vi "AlliGator Python Plugin Data to Graph v1.1.vi"(7 "AlliGator Ctrl Refnums":T8, 8 "error in (no error)":errorcluster, 10 "Output Destination":string, 11 "Plugin_Data":T1) -> (0 "error out":errorcluster, 3 "Message":string)   [LabVIEW 2021, in "AlliGator Python Plugins.lvlib"]
uses:
  AlliGator Python Plugins.lvlib
  Strings/Strings.lvlib
  GUI/AlliGator GUI.lvlib
  Graphs/XY Graph/XY Graph Add-Ons.lvlib
  GUI/AlliGator Registered Events Ctrl Refnums.ctl
  Source Image/AlliGator Displayed Image.ctl
  Source Image/AlliGator Source Image.lvlib
  GUI/AlliGator Dataset Ctrl Refnums.ctl
  Phasor/Phasor Calibration Type.ctl
  Phasor/Phasor.lvlib
  GUI/AlliGator Phasor Graph Ctrl Refnums.ctl
  GUI/AlliGator Phasor Plot Ctrl Refnums.ctl
  GUI/AlliGator State Indicator.ctl
  GUI/AlliGator Main Window Tabs.ctl
  GUI/AlliGator Other Ctrl Refnums.ctl
  Histograms/Histogram Bin Position.ctl
  Histograms/Histogram Window.lvlib
  Histograms/Histogram Bin Option.ctl
  Histograms/Linear Histogram Options.ctl
  GUI/AlliGator Image Histogram Control Refnums.ctl
  Fits/IRF(X)PSED/Decay Fit Parameters & Derived Quantities List v2.ctl
  Fits/Fits.lvlib
  Decay Fit Parameter Map/AlliGator Decay Fit Map Control Refnums.ctl
  Decay Fit Parameter Map/AlliGator Decay Fit Parameter Map.lvlib
  Parameter Map/AlliGator Parameter Map Control Refnums.ctl
  Parameter Map/AlliGator Parameter Map.lvlib
  GUI/AlliGator Ctrl Refnums.ctl
  API v1/AlliGator Python Plugin Image Data v1.ctl
  AlliGator Python Plugin FLI Dataset Data v1.1.ctl
  Image/Image Point.ctl
  Image/Image.lvlib
  AlliGator Python Plugin Parameter Map Data v1.1.ctl
  API v1/AlliGator Python Plugin Plot Data v1.ctl
  API v1/AlliGator Python Plugin Graph Data v1.ctl
  AlliGator Python Plugin Data v1.1.ctl
panel:
  # "see the License on the block diagram (Ctrl+E or Window:Show Block Diagram)"
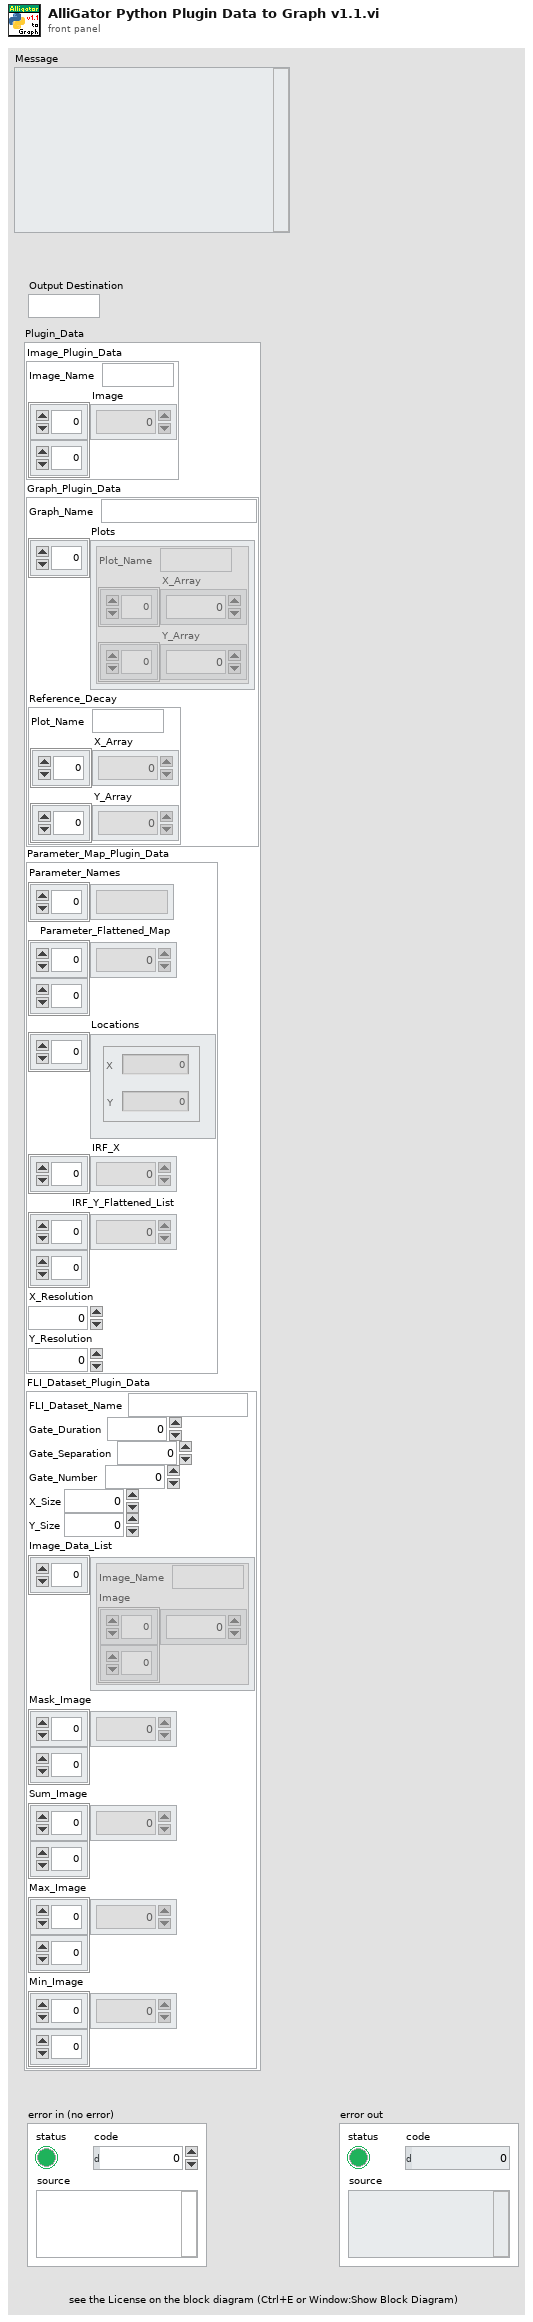
[diagram p1: front panel]
types:
  T1 = typedef "AlliGator Python Plugins.lvlib/AlliGator Python Plugin Data v1.1.ctl" = cluster{"Image_Plugin_Data":T2, "Graph_Plugin_Data":T3, "Parameter_Map_Plugin_Data":T5, "FLI_Dataset_Plugin_Data":T7}
  T2 = typedef "AlliGator Python Plugins.lvlib/AlliGator Python Plugin Image Data v1.ctl" = cluster{"Image_Name":string, "Image":sgl[][]}
  T3 = typedef "AlliGator Python Plugins.lvlib/AlliGator Python Plugin Graph Data v1.ctl" = cluster{"Graph_Name":string, "Plots":T4[], "Reference_Decay":T4}
  T4 = typedef "AlliGator Python Plugins.lvlib/AlliGator Python Plugin Plot Data v1.ctl" = cluster{"Plot_Name":string, "X_Array":dbl[], "Y_Array":dbl[]}
  T5 = typedef "AlliGator Python Plugins.lvlib/AlliGator Python Plugin Parameter Map Data v1.1.ctl" = cluster{"Parameter_Names":string[], "Parameter_Flattened_Map":dbl[][], "Locations":T6[], "IRF_X":dbl[], "IRF_Y_Flattened_List":dbl[][], "X_Resolution":i32, "Y_Resolution":i32}
  T6 = typedef "Image.lvlib/Image Point.ctl" = cluster{"X":i32, "Y":i32}
  T7 = typedef "AlliGator Python Plugins.lvlib/AlliGator Python Plugin FLI Dataset Data v1.1.ctl" = cluster{"FLI_Dataset_Name":string, "Gate_Duration":dbl, "Gate_Separation":dbl, "Gate_Number":i32, "X_Size":i32, "Y_Size":i32, "Image_Data_List":T2[], "Mask_Image":u16[][], "Sum_Image":sgl[][], "Max_Image":sgl[][], "Min_Image":sgl[][]}
  T8 = typedef "AlliGator GUI.lvlib/AlliGator Ctrl Refnums.ctl" = cluster{"Other AlliGator Ctrl Refnums":T9, "Phasor Plot Ctrl Refnums":T10, "Phasor Graph Ctrl Refnums":T11, "Dataset Control Refnums":T12, "Registered Events Ctrl Refnums":T13, "Image Histogram Ctrl Refnums":T14, "Decay Fit Map Ctrl Refnums":T15, "Parameter Map Ctrl Refnums":T16}
  T9 = typedef "AlliGator GUI.lvlib/AlliGator Other Ctrl Refnums.ctl" = cluster{"State Indicators":refnum<vi>, " Progress Bar":refnum<vi>, "Decay Graph Active":refnum<vi>, "Decay Statistics Bin":refnum<vi>, "Time Step":refnum<vi>, "Use File Timestamp":refnum<vi>, "Tab Control":refnum<vi>, "CPU":refnum<vi>, "Abort Fit":refnum<vi>, "Dataset File/Folder Path":refnum<vi>, "Abort ROI Creation":refnum<vi>, "Event LED":refnum<vi>, "Dataset File/Folder Path 2":refnum<vi>, "Dataset File/Folder Path 3":refnum<vi>, "Dataset File/Folder Path 4":refnum<vi>, "Dataset File/Folder Path 5":refnum<vi>, "Dataset File/Folder Path 6":refnum<vi>, "Dataset File/Folder Path 7":refnum<vi>, "Dataset File/Folder Path 8":refnum<vi>, "Dataset File/Folder Path 9":refnum<vi>, "Dataset File/Folder Path 10":refnum<vi>, "Dataset File/Folder Path 11":refnum<vi>}
  T10 = typedef "AlliGator GUI.lvlib/AlliGator Phasor Plot Ctrl Refnums.ctl" = cluster{"Phasor Ratio":refnum<vi>, "Modulus Lifetime":refnum<vi>, "Phasor at cursor (m, phi)":refnum<vi>, "Phase Lifetime":refnum<vi>, "Phasor at cursor (g, s)":refnum<vi>, "Phasor Plor Average Lifetime":refnum<vi>, "Phasor Plot Active":refnum<vi>, "Save Phasor Plot":refnum<vi>, "Image Overlay Color":refnum<vi>, "Phasor Plot Color Scale":refnum<vi>, "Reference 1 Button":refnum<vi>, "Reference 2 Button":refnum<vi>, "True Phasor Plot Value":refnum<vi>}
  T11 = typedef "AlliGator GUI.lvlib/AlliGator Phasor Graph Ctrl Refnums.ctl" = cluster{"Phasor Ratio":refnum<vi>, "Modulus Lifetime":refnum<vi>, "Phasor at cursor (m, phi)":refnum<vi>, "Phase Lifetime":refnum<vi>, "Phasor at cursor (g, s)":refnum<vi>, "Phasor Graph Average Lifetime":refnum<vi>, "Phasor Graph Active":refnum<vi>, "Save Phasor Graph":refnum<vi>, "Phasor Frame Slide":refnum<vi>, "Single Step Phasor":refnum<vi>, "Calibration Type":refnum<vi>, "Show Line":refnum<vi>, "Phase Lifetime 1":refnum<vi>, "Phase Lifetime 2":refnum<vi>, "Phasor Graph Frequency":refnum<vi>, "Phasor Reference 1 Control":refnum<vi>, "Phasor Reference 2 Control":refnum<vi>, "Calibration Lifetime":refnum<vi>, "Phase Lifetime SDV":refnum<vi>, "Average Lifetime SDV":refnum<vi>, "Phasor Ratio SDV":refnum<vi>, "Modulus Lifetime SDV":refnum<vi>}
  T12 = typedef "AlliGator GUI.lvlib/AlliGator Dataset Ctrl Refnums.ctl" = cluster{"Current Data":refnum<vi>, "Gate Image Slide":refnum<vi>, "Time Point Slide":refnum<vi>, "Current Time Stamp":refnum<vi>, "Save Image":refnum<vi>, "Displayed Image":refnum<vi>, "Overlay Mode":refnum<vi>, "Phasor Overlay Color":refnum<vi>, "Image Color Scale":refnum<vi>, "Use ROI as Search Area":refnum<vi>, "Source Image ROI Color":refnum<vi>, "True Pixel Value":refnum<vi>}
  T13 = typedef "AlliGator GUI.lvlib/AlliGator Registered Events Ctrl Refnums.ctl" = cluster{"Time Point Slider":refnum<vi>, "Phasor Plot Display Range":refnum<vi>, "Decay Graph":refnum<vi>, "Decay Statistics Graph":refnum<vi>, "Intensity Time Trace":refnum<vi>, "Phasor Graph":refnum<vi>, "Phasor Ratio Graph":refnum<vi>, "Lifetime Graph":refnum<vi>, "Phasor Plot Display":refnum<vi>, "Source Image Display":refnum<vi>, "Decay Fit Parameter Map Display Range":refnum<vi>, "Decay Fit Parameter Map Display":refnum<vi>, "Parameter Map Display Range":refnum<vi>, "Parameter Map Display":refnum<vi>, "Phasor Plot Display Range":refnum<vi>}
  T14 = typedef "AlliGator GUI.lvlib/AlliGator Image Histogram Control Refnums.ctl" = cluster{"Image Histogram":refnum<vi>, "Image Histogram Options":refnum<vi>, "Image Histogram Active":refnum<vi>, "Image Histogram Upper Percentile":refnum<vi>, "Image Histogram Lower Percentile":refnum<vi>, "Auto-Adjust Contrast":refnum<vi>}
  T15 = typedef "AlliGator Decay Fit Parameter Map.lvlib/AlliGator Decay Fit Map Control Refnums.ctl" = cluster{"Decay Fit Parameter Map Color Scale":refnum<vi>, "Decay Fit Parameter":refnum<vi>, "Max Parameter":refnum<vi>, "Min Parameter":refnum<vi>, "Decay Fit Parameter Map Display":refnum<vi>, "Decay Fit Parameter Map Display Range":refnum<vi>, "Decay Parameter Map X":refnum<vi>, "Decay Parameter Map Y":refnum<vi>, "Decay Parameter Map Value":refnum<vi>}
  T16 = typedef "AlliGator Parameter Map.lvlib/AlliGator Parameter Map Control Refnums.ctl" = cluster{"Parameter Map Color Scale":refnum<vi>, "Map Parameter":refnum<vi>, "Max Parameter":refnum<vi>, "Min Parameter":refnum<vi>, "Parameter Map Display":refnum<vi>, "Parameter Map Display Range":refnum<vi>, "Parameter Map Set":refnum<vi>, "Parameter Map X":refnum<vi>, "Parameter Map Y":refnum<vi>, "Parameter Map Value":refnum<vi>}
  T17 = typedef "XY Graph Add-Ons.lvlib/XY Graph Refnum.ctl" = refnum<vi>
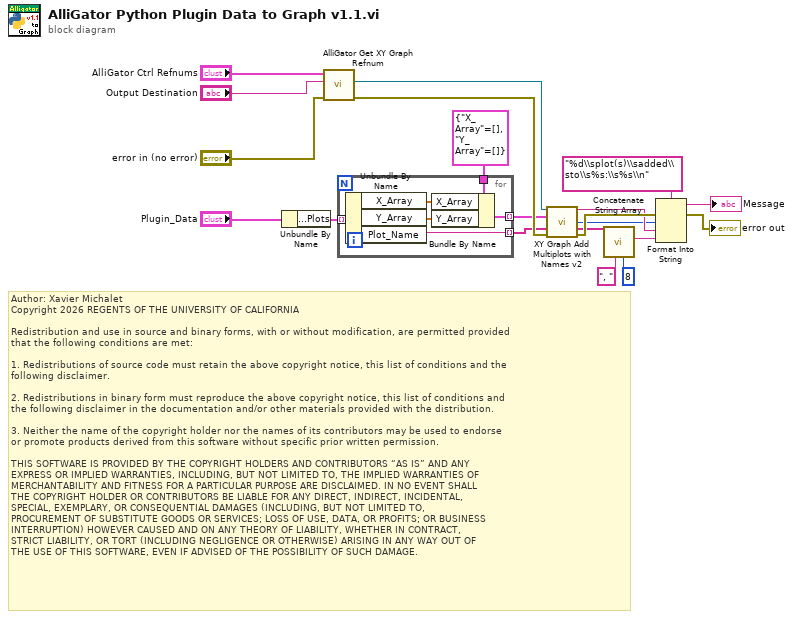
[diagram p0: block diagram]
diagram:
  # "Author: Xavier Michalet\nCopyright 2026 REGENTS OF THE UNIVERSITY OF CALIFORNIA\n\nRedistribution and use in source and binary forms, with or without modification, are permitted provided\nthat the following conditions are met:\n\n1. Redistributions of source code must retain the above copyright notice, this list of conditions and the\nfollowing disclaimer.\n\n2. Redistributions in binary form must reproduce the above copyright notice, this list of conditions and\nthe following disclaimer in the documentation and/or other materials provided with the distribution.\n\n3. Neither the name of the copyright holder nor the names of its contributors may be used to endorse \nor promote products derived from this software without specific prior written permission.\n\nTHIS SOFTWARE IS PROVIDED BY THE COPYRIGHT HOLDERS AND CONTRIBUTORS “AS IS” AND ANY \nEXPRESS OR IMPLIED WARRANTIES, INCLUDING, BUT NOT LIMITED TO, THE IMPLIED WARRANTIES OF\nMERCHANTABILITY AND FITNESS FOR A PARTICULAR PURPOSE ARE DISCLAIMED. IN NO EVENT SHALL\nTHE COPYRIGHT HOLDER OR CONTRIBUTORS BE LIABLE FOR ANY DIRECT, INDIRECT, INCIDENTAL, \nSPECIAL, EXEMPLARY, OR CONSEQUENTIAL DAMAGES (INCLUDING, BUT NOT LIMITED TO, \nPROCUREMENT OF SUBSTITUTE GOODS OR SERVICES; LOSS OF USE, DATA, OR PROFITS; OR BUSINESS\nINTERRUPTION) HOWEVER CAUSED AND ON ANY THEORY OF LIABILITY, WHETHER IN CONTRACT, \nSTRICT LIABILITY, OR TORT (INCLUDING NEGLIGENCE OR OTHERWISE) ARISING IN ANY WAY OUT OF\nTHE USE OF THIS SOFTWARE, EVEN IF ADVISED OF THE POSSIBILITY OF SUCH DAMAGE."
  n1 = Unbundle By Name("Plugin_Data") -> ("Graph_Plugin_Data.Plots"=w8:T4[])
  n2 = call "AlliGator Get XY Graph Refnum.vi"("error in (no error)"="error in (no error)", "XY Graph Name"="Output Destination", "AlliGator Ctrl Refnums"="AlliGator Ctrl Refnums") -> ("error out"=w17:errorcluster, "XY Graph reference"=w19:T17)  [unwired: 7 in]
  n3 = for {
    tunnel: w8 -> [w26] mode=indexing
    tunnel: [w25] -> w3 mode=indexing
    tunnel: cluster{"X_Array":dbl[], "Y_Array":dbl[]} {"X_Array"=[], "Y_Array"=[]} -> [w23]
    tunnel: [w21] -> w2 mode=indexing
    n4 = Unbundle By Name(w26) -> ("X_Array"=w24:dbl[], "Y_Array"=w22:dbl[], "Plot_Name"=w25:string)
    n5 = Bundle By Name(cluster=w23, "X_Array"=w24, "Y_Array"=w22) -> (w21:cluster{"X_Array":dbl[], "Y_Array":dbl[]})
  }
  n6 = call "XY Graph Add Multiplots with Names v2.vi"("XYGraph in"=w19, "Array of Plots"=w2, "Array of Plot Names (\"Plot\")"=w3, "error in (no error)"=w17) -> ("XY Graph Caption (or Label)"=w11:string, "Number of Plots Added"=w10:i32, "Added Plot Names"=w4:string[], "error out"=w13:errorcluster)  [unwired: 7 in, 1 out]
  n7 = call "Concatenate String Array.vi"("Max Number of Elements (None: -1)"=8, "Separator (TAB)"=", ", "String Array"=w4) -> ("Formatted String"=w12:string)  [unwired: 8 in]
  n8 = Format Into String(format string="%d\\splot(s)\\sadded\\sto\\s%s:\\s%s\\n", error in=w13, w10, w11, w12) -> (resulting string=→"Message":string, error out=→"error out":errorcluster)  [unwired: 1 in]
